vi "String to Array.vi"(0 "Input String":string=" 12, 213, 26") -> (1 "Array of Strings":string[](array[string]), 2 "Array of Numbers":i32[](array[numeric]))   [LabVIEW 2017]
panel:
  # "This VI takes a comma-\ndelimted string input and converts it to an array of strings and an array of numbers."
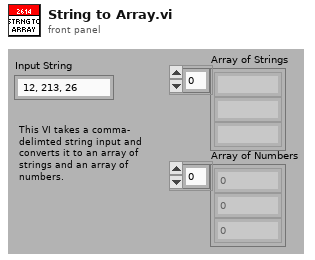
[diagram p1: front panel]
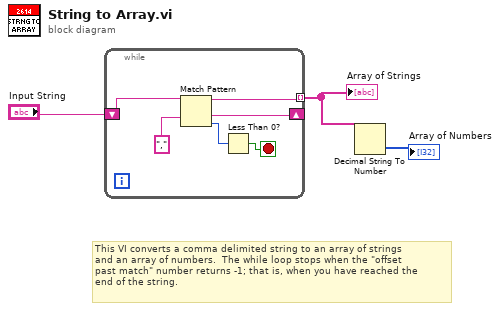
[diagram p0: block diagram]
diagram:
  # "This VI converts a comma delimited string to an array of strings \nand an array of numbers.  The while loop stops when the \"offset\npast match\" number returns -1; that is, when you have reached the \nend of the string."
  n1 = while {
    tunnel: [w6] -> w2 mode=indexing
    shift-right: [w7] -> _
    shift-left: "Input String" -> [w9]
    stop <- w4 stop-if-true
    n2 = Match Pattern(string=w9, regular expression=",") -> (before substring=w6:string, after substring=w7:string, offset past match=w5:i32)  [unwired: 2 out]
    n3 = Less Than 0?(x=w5) -> (x < 0?=w4:bool)
  }
  "Array of Strings" <- w2
  n4 = Decimal String To Number(string=w2) -> (number=→"Array of Numbers":i32[])  [unwired: 3 out]
